vi "manager.create.vi"(8 "error in (no error)":errorcluster, 11 "LabVIEW-MIDI-XPLAT in":refnum<class "LabVIEW-MIDI-XPLAT.lvclass">) -> (0 "error out":errorcluster, 3 "LabVIEW-MIDI-XPLAT out":refnum<class "LabVIEW-MIDI-XPLAT.lvclass">)   [LabVIEW 2020, in "LabVIEW-MIDI-XPLAT.lvclass"]
uses:
  LabVIEW-MIDI-XPLAT.lvclass
  LabVIEW-MIDI-XPLAT.lvclass/LabVIEW-MIDI-XPLAT.ctl
  target/release/midi_driver.dll
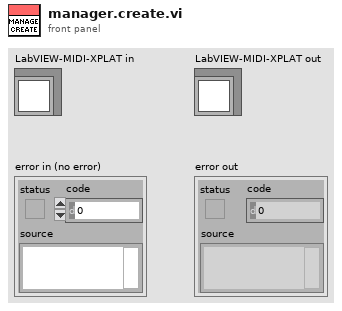
[diagram p1: front panel]
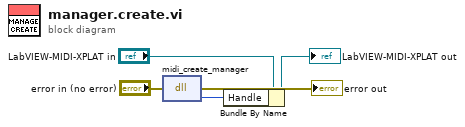
[diagram p0: block diagram]
diagram:
  n1 = dll-call lib="C:/code/LabVIEW-MIDI-XPLAT/target/release/midi_driver.dll" fn="midi_create_manager"(error in="error in (no error)") -> (error out=→"error out":errorcluster, "Handle"=w3:i32)  [unwired: 2 in, 1 out]
  n2 = Bundle By Name(cluster="LabVIEW-MIDI-XPLAT in", "Handle"=w3) -> (→"LabVIEW-MIDI-XPLAT out":refnum<class "LabVIEW-MIDI-XPLAT.lvclass">)
